vi "Main_XXa.vi"() -> ()   [LabVIEW 2020]
panel:
  out "sum":i32
  in  "Puzzle":string
  in  "Example":string
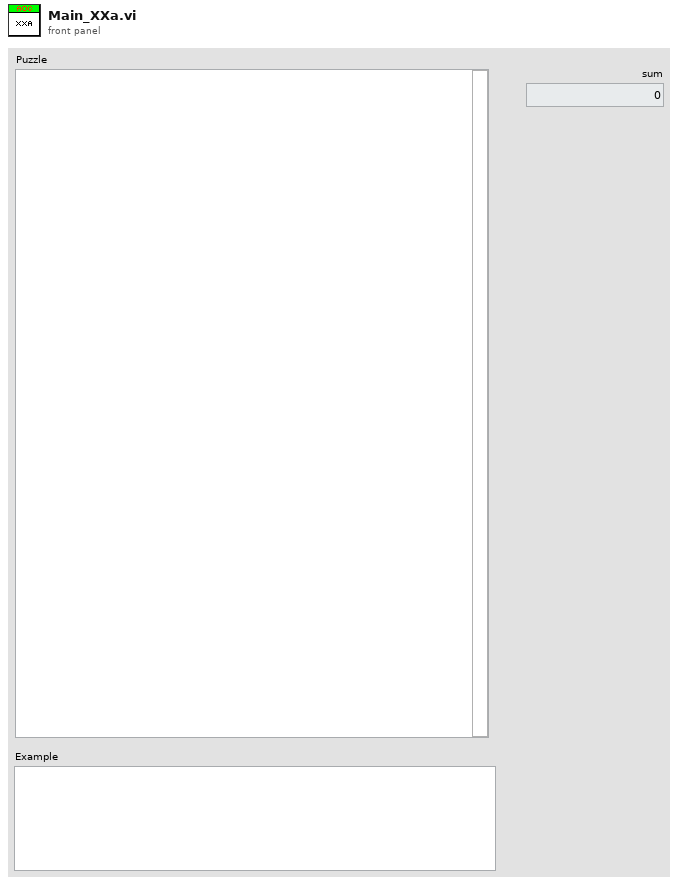
[diagram p1: front panel]
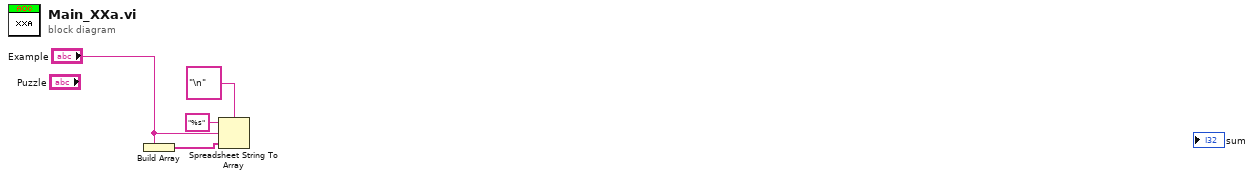
[diagram p0: block diagram]
diagram:
  n1 = Build Array("Example") -> (w4:string[])
  n2 = Spreadsheet String To Array(delimiter (Tab)="\n", format string="%s", spreadsheet string="Example", array type (2D Dbl)=w4) -> ()  [unwired: 1 out]
